vi "GetAnalogOutValues.vi"(8 "error in (no error)":errorcluster caption="Fehler (Eingang, kein Fehler)", 11 "lLSID":i32) -> (0 "error out":errorcluster caption="error in (no error)", 2 "AnaOut2":i32, 3 "Anaout1":i32)   [LabVIEW 2015]
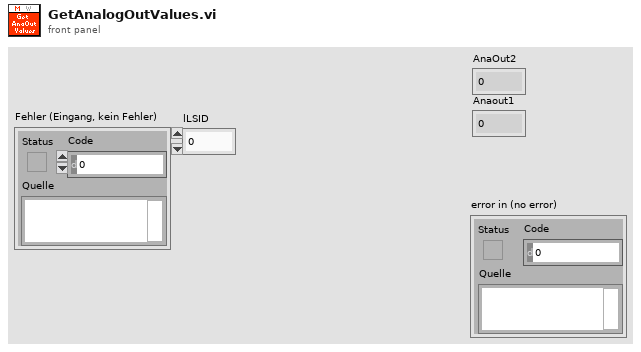
[diagram p1: front panel]
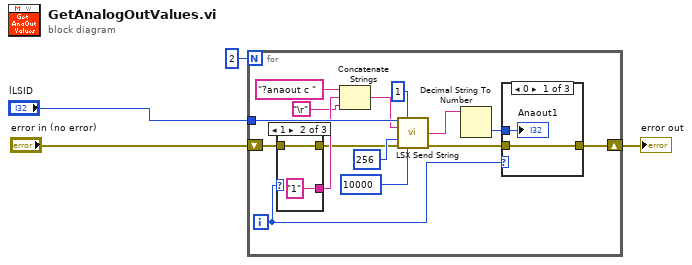
[diagram p0: block diagram]
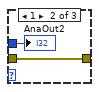
[diagram p2: hidden frame]
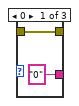
[diagram p4: hidden frame]
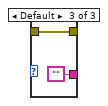
[diagram p5: hidden frame]
diagram:
  n1 = for {
    N: 2 -> [_]
    tunnel: "lLSID" -> [w19]
    shift-right: [w10] -> w1
    shift-left: "error in (no error)" -> [w9]
    i -> [w12]
    n2 = case shown="1" w12 {
      tunnel: ["0" "1" ""] -> w14
      tunnel: [w25 w27 w29] -> w8
      tunnel: w9 -> [w25 w27 w29]
      frame 0 {
      }
      frame 1 {
      }
      frame Default {
      }
    }
    n3 = Concatenate Strings("?anaout c ", w14, "\r") -> (w13:string)
    n4 = call "LSX Send String.vi"("lLSID"=w19, "bReadLine"=1, "pcStr"=w13, "lMaxLen"=256, "error in (no error)"=w8, "lTimeOut"=10000) -> ("pcRet out"=w7:string, "error out"=w11:errorcluster)  [unwired: 6 in, 2 out]
    n5 = Decimal String To Number(string=w7) -> (number=w6:i32)  [unwired: 2 in, 1 out]
    n6 = case shown="0" w12 {
      tunnel: w6 -> [w20 w22 _]
      tunnel: w11 -> [w21 w23 w24]
      tunnel: [w21 w23 w24] -> w10
      frame 0 {
        "Anaout1" <- w20
      }
      frame 1 {
        "AnaOut2" <- w22
      }
      frame Default {
      }
    }
  }
  "error out" <- w1
